vi "Rebuild Command Table.vi"   [LabVIEW 2019, in "LINXx.lvlib"]
doc: "Dev helper to automatically generate table of command codes from the base LinxListener code"
uses:
  LINXx.lvlib
  <vilib>/regexp/Match Regular Expression.xnode
types:
  T1 = enum16{"Native", "Native Command Line", "UNIX", "Macintosh", "DOS"}
  T2 = enum16{"open", "replace", "create", "open or create", "replace or create", "replace or create with confirmation"}
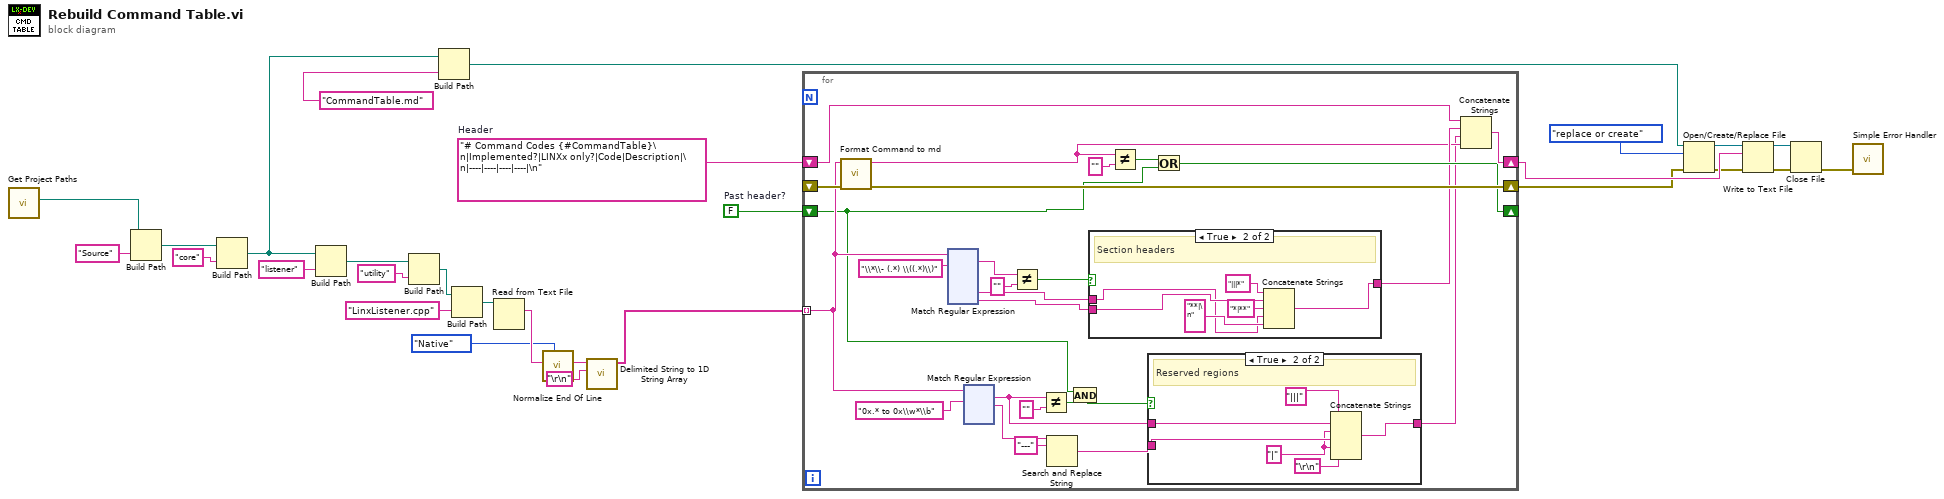
[diagram p0: block diagram]
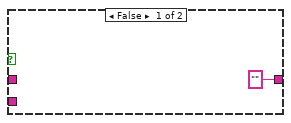
[diagram p2: hidden frame]
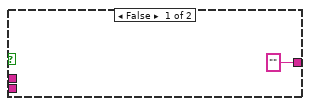
[diagram p3: hidden frame]
diagram:
  w17 = FALSE  # Past header?
  w18 = "# Command Codes {#CommandTable}\n|Implemented?|LINXx only?|Code|Description|\n|----|----|----|----|\n"  # Header
  n1 = call "Get Project Paths.vi"() -> ("Firmware path"=w19:path)  [unwired: 8 in, 3 out]
  n2 = Build Path(base path=w19, name or relative path="Source") -> (appended path=w2:path)
  n3 = Build Path(base path=w2, name or relative path="core") -> (appended path=w1:path)
  n4 = Build Path(base path=w1, name or relative path="listener") -> (appended path=w24:path)
  n5 = Build Path(base path=w24, name or relative path="utility") -> (appended path=w22:path)
  n6 = Build Path(base path=w1, name or relative path="CommandTable.md") -> (appended path=w10:path)
  n7 = Build Path(base path=w22, name or relative path="LinxListener.cpp") -> (appended path=w21:path)
  n8 = Read from Text File(file (use dialog)=w21) -> (text=w7:string)  [unwired: 3 in, 3 out]
  n9 = call <vilib>:"Normalize End Of Line.vi"("end of line (Native)"=T1."Native", "string in"=w7) -> ("string out"=w5:string)  [unwired: 6 in]
  n10 = call <vilib>:"Delimited String to 1D String Array.vi"("delimiter"="\r\n", "delimited string"=w5) -> ("string array"=w6:string[])  [unwired: 9 in]
  n11 = for {
    tunnel: w6 -> [w41] mode=indexing
    shift-right: [w53] -> w15
    shift-left: w18 -> [w54]
    shift-right: [w51] -> w11
    shift-left: _ -> [w52]
    shift-right: [w44] -> _
    shift-left: w17 -> [w30]
    n12 = call "Format Command to md.vi"("error in (no error)"=w52, "line"=w41) -> ("error out"=w51:errorcluster, ".md table row"=w42:string)  [unwired: 7 in, 1 out]
    n13 = xnode "Match Regular Expression"("input string"=w41, "regular expression"="\\*\\- (.*) \\((.*)\\)") -> ("whole match"=w49:string, "submatch 1"=w47:string, "submatch 2"=w32:string)  [unwired: 4 in, 4 out]
    n14 = xnode "Match Regular Expression"("input string"=w41, "regular expression"="0x.* to 0x\\w*\\b") -> ("whole match"=w36:string, "after match"=w34:string)  [unwired: 4 in, 3 out]
    n15 = Not Equal?(x=w49, y="") -> (x != y?=w29:bool)
    n16 = Not Equal?(x=w36, y="") -> (x != y?=w39:bool)
    n17 = Search and Replace String(input string=w34, search string="---") -> (result string=w35:string)  [unwired: 6 in, 3 out]
    n18 = And(x=w30, y=w39) -> (x .and. y?=w31:bool)
    n19 = case shown="True" w29 {
      tunnel: w47 -> [_ w177]
      tunnel: ["" w181] -> w43
      tunnel: w32 -> [_ w180]
      frame False {
      }
      frame True {
        # "Section headers"
        n20 = Concatenate Strings("|||*" ("string"), w180, "*|**" ("string"), w177, "**|\n" ("string")) -> (w181:string)
      }
    }
    n21 = Not Equal?(x=w42, y="") -> (x != y?=w45:bool)
    n22 = case shown="True" w31 {
      tunnel: w36 -> [_ w61]
      tunnel: ["" w60] -> w37
      tunnel: w35 -> [_ w59]
      frame False {
      }
      frame True {
        w57 = "|" ("string")
        # "Reserved regions"
        n23 = Concatenate Strings("|||" ("string"), w61, w57, w59, w57, "\r\n") -> (w60:string)
      }
    }
    n24 = Or(x=w45, y=w30) -> (x .or. y?=w44:bool)
    n25 = Concatenate Strings(w54, w43, w37, w42) -> (w53:string)
  }
  n26 = Open/Create/Replace File(file path (use dialog)=w10, error in=w11, operation (0:open)=T2."replace or create") -> (refnum out=w13:refnum<file>, error out=w14:errorcluster)  [unwired: 3 in, 1 out]
  n27 = Write to Text File(file (use dialog)=w13, text=w15, error in=w14) -> (refnum out=w12:refnum<file>, error out=w16:errorcluster)  [unwired: 1 in, 1 out]
  n28 = Close File(refnum=w12, error in=w16) -> (error out=w8:errorcluster)  [unwired: 1 out]
  n29 = call <vilib>:"Simple Error Handler.vi"("error in (no error)"=w8) -> ()  [unwired: 4 in, 5 out]
